vi "test-new-clock.vi"() -> ()   [LabVIEW 2019]
uses:
  <vilib>/Rock Robotics/WPI/ThirdParty/JAS_Junk/TrajLib/Trajectory_Library.lvlib
panel:
  out "OS Clock":dbl format="%35.6f"
  out "Waveform Chart":cluster{"FPGA_Time_Seconds":dbl, dbl, dbl}(graph)
  out "Error Count":i32
  out "Loop Count":i32
  out "FPGA Clock":dbl format="%35.6f"
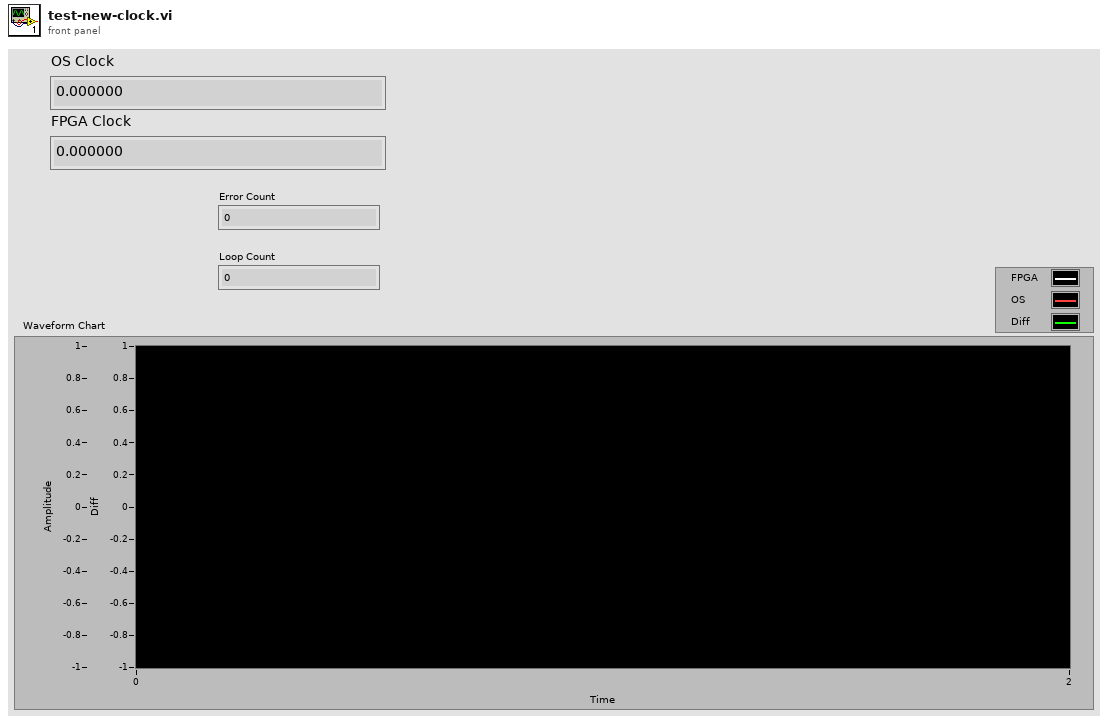
[diagram p1: front panel]
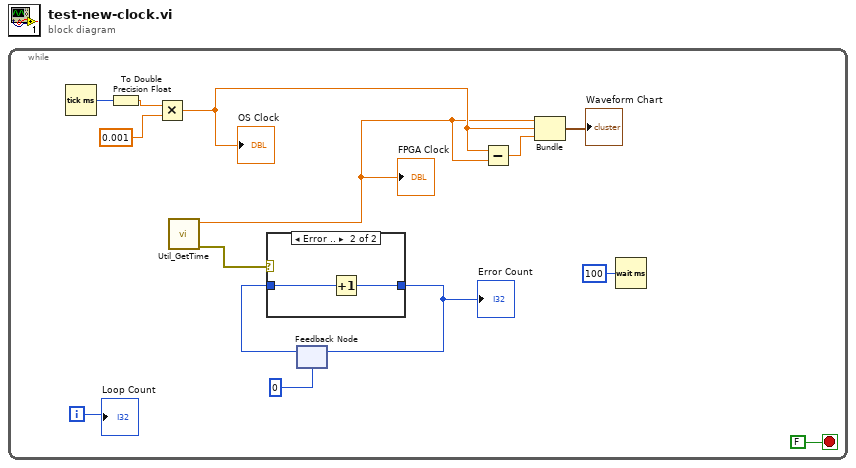
[diagram p0: block diagram]
diagram:
  n1 = while {
    i -> [w13]
    stop <- FALSE stop-if-true
    n2 = Tick Count (ms)() -> (millisecond timer value=w7:u32)
    n3 = To Double Precision Float(number=w7) -> (double precision float=w6:dbl)
    n4 = Multiply(x=w6, y=0.001) -> (x*y=w4:dbl)
    "OS Clock" <- w4
    n5 = call <vilib>:"Util_GetTime.vi"() -> ("error out"=w1:errorcluster, "FPGA_Time_Seconds"=w2:dbl)  [unwired: 10 in]
    "FPGA Clock" <- w2
    n6 = feedback #1(0) -> (w11:i32)
    n7 = case shown="Error .." w1 {
      tunnel: w11 -> [w15 w16]
      tunnel: [w15 w17] -> w10
      frame No Error {
      }
      frame Error {
        n8 = Increment(x=w16) -> (x+1=w17:i32)
      }
    }
    "Error Count" <- w10
    n9 = feedback-in #1(w10) -> ()
    n10 = Subtract(x=w4, y=w2) -> (x-y=w3:dbl)
    n11 = Bundle("FPGA_Time_Seconds"=w2, w4, w3) -> (→"Waveform Chart":cluster{"FPGA_Time_Seconds":dbl, dbl, dbl})  [unwired: 1 in]
    n12 = Wait (ms)(milliseconds to wait=u32 100) -> ()  [unwired: 1 out]
    "Loop Count" <- w13
  }
